vi "bt_read.vi"(10 "Packet Size":i32, 11 "Received Bytes":string) -> (0 "Jitter":i32, 1 "Received Message Count":i32, 2 "Received Bytes Size":i32, 3 "Raw Data":sgl[](array[numeric]))   [LabVIEW 2023]
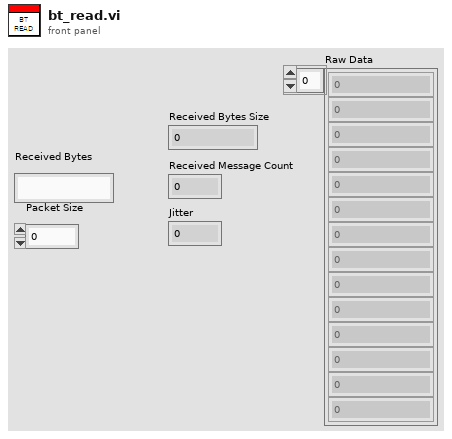
[diagram p1: front panel]
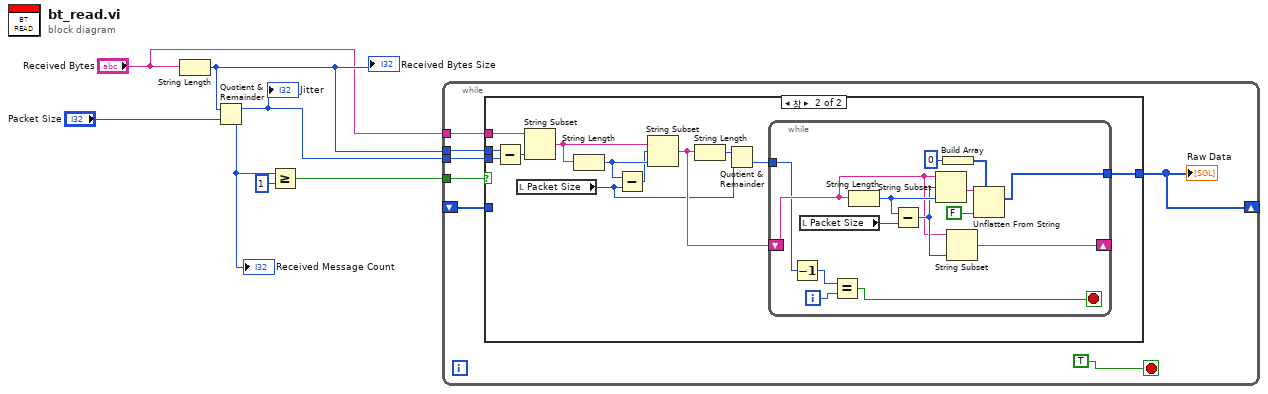
[diagram p0: block diagram]
diagram:
  n1 = String Length(string="Received Bytes") -> (length=w3:i32)
  "Received Bytes Size" <- w3
  n2 = Quotient & Remainder(x=w3, y="Packet Size") -> (x-y*floor(x/y)=w4:i32, floor(x/y)=w7:i32)
  "Jitter" <- w4
  "Received Message Count" <- w7
  n3 = Greater Or Equal?(x=w7, y=1) -> (x >= y?=w5:bool)
  n4 = while {
    tunnel: w5 -> [w14]
    tunnel: w4 -> [w13]
    tunnel: w3 -> [w12]
    tunnel: "Received Bytes" -> [w11]
    shift-right: [w9] -> _
    shift-left: _ -> [w8]
    stop <- TRUE stop-if-true
    n5 = case shown="참" w14 {
      tunnel: w11 -> [_ w27]
      tunnel: w12 -> [_ w26]
      tunnel: w13 -> [_ w25]
      tunnel: [w15 w16] -> w9
      tunnel: w8 -> [w15 _]
      frame False {
      }
      frame True {
        n6 = Subtract(x=w26, y=w25) -> (x-y=w24:i32)
        n7 = local read "Packet Size"() -> (w18:i32)
        n8 = String Subset(string=w27, length (rest)=w24) -> (substring=w19:string)  [unwired: 1 in]
        n9 = String Length(string=w19) -> (length=w23:i32)
        n10 = Subtract(x=w23, y=w18) -> (x-y=w22:i32)
        n11 = String Subset(string=w19, offset (0)=w22, length (rest)=w23) -> (substring=w20:string)
        n12 = String Length(string=w20) -> (length=w21:i32)
        n13 = Quotient & Remainder(x=w21, y=w18) -> (floor(x/y)=w17:i32)  [unwired: 1 out]
        n14 = while {
          shift-right: [w39] -> _
          shift-left: w20 -> [w38]
          tunnel: w17 -> [w32]
          tunnel: [w28] -> w16
          i -> [w30]
          stop <- w29 stop-if-true
          n15 = Decrement(x=w32) -> (x-1=w31:i32)
          n16 = local read "Packet Size"() -> (w33:i32)
          n17 = Equal?(x=w31, y=w30) -> (x = y?=w29:bool)
          n18 = String Length(string=w38) -> (length=w41:i32)
          n19 = Subtract(x=w41, y=w33) -> (x-y=w40:i32)
          n20 = String Subset(string=w38, offset (0)=w40, length (rest)=w41) -> (substring=w37:string)
          n21 = Build Array(0 ("원소")) -> (w34:i32[])
          n22 = String Subset(string=w38, length (rest)=w40) -> (substring=w39:string)  [unwired: 1 in]
          n23 = Unflatten From String(type=w34, binary string=w37, data includes array or string size? (T)=FALSE ("데이터가 배열 또는 문자열 크기를 포함? (참)")) -> (value=w28:i32[])  [unwired: 2 in, 2 out]
        }
      }
    }
    "Raw Data" <- w9
  }
